vi "Set BBM Vacuum.vi"(6 "On/Off":bool, 8 "error in (no error)":errorcluster, 9 "Slot Number":u32, 10 "Chuck Number":u32, 11 "Gantry Class in":refnum<class "Gantry Class.lvclass">) -> (0 "error out":errorcluster, 3 "Gantry Class out":refnum<class "Gantry Class.lvclass">)   [LabVIEW 2011, in "Gantry Class.lvclass"]
uses:
  Gantry Class.lvclass
  WorkTable Class/WorkTable Class.lvclass
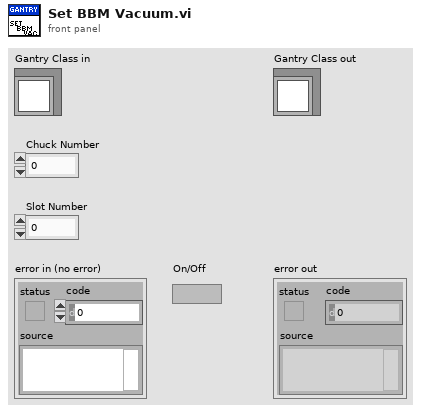
[diagram p1: front panel]
types:
  T1 = typedef "Worktable_BBM Slot.ctl" = cluster{"BBM Slot State":enum16{"Empty", "Unglued", "Stamped", "PartOnTop", "Weighted", "Unpotted", "Potted"}, "BBM Type":enum16{"BBM", "GlassSlide"}, "HDI Type":enum16{"HDI", "Polyimide"}, "Vacuum Channel":u8, "Location/Orientation BBM":T2, "Location/Orientation HDI":T2}
  T2 = typedef "Position_Orientation.ctl" = cluster{"Center":refnum<class "Vec3d Class.lvclass">, "Orientation":refnum<class "Orient3d Class.lvclass">}
  T3 = cluster{"BBM Chucks":cluster{"BBM Slots":T1[]}[]}
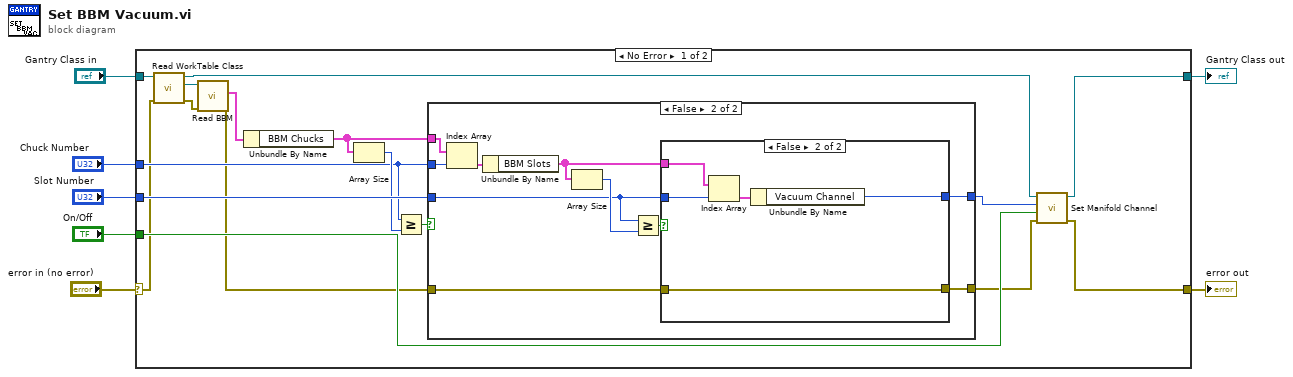
[diagram p0: block diagram]
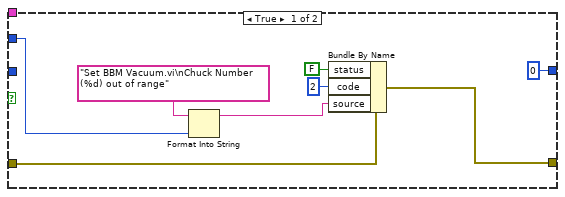
[diagram p2: hidden frame]
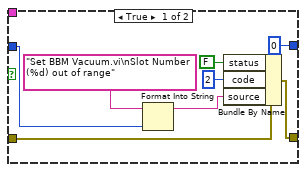
[diagram p3: hidden frame]
diagram:
  n1 = case shown="No Error" "error in (no error)" {
    selector: "error in (no error)" -> [w9 w57]
    tunnel: [w11 w57] -> w6
    tunnel: [w12 w56] -> w4
    tunnel: "Gantry Class in" -> [w24 w56]
    tunnel: "Chuck Number" -> [w18 _]
    tunnel: "Slot Number" -> [w21 _]
    tunnel: "On/Off" -> [w15 _]
    frame No Error {
      n2 = call-dynamic "Read WorkTable Class.vi"("error in"=w9, "Gantry Class in"=w24) -> ("error out"=w10:errorcluster, "WorkTable Class.lvclass"=w23:refnum<class "WorkTable Class.lvclass">, "Gantry Class out"=w13:refnum<class "Gantry Class.lvclass">)  [unwired: 7 in]
      n3 = call-dynamic "Read BBM.vi"("error in (no error)"=w10, "WorkTable Class in"=w23) -> ("error out"=w8:errorcluster, "BBM"=w22:T3)  [unwired: 7 in, 1 out]
      n4 = Unbundle By Name(w22) -> ("BBM Chucks"=w20:cluster{"BBM Slots":T1[]}[])
      n5 = Array Size(array=w20) -> (size(s)=w19:i32)
      n6 = Greater Or Equal?(x=w18, y=w19) -> (x >= y?=w17:bool)
      n7 = case shown="False" w17 {
        tunnel: w18 -> [w28 w42]
        tunnel: w21 -> [_ w36]
        tunnel: w20 -> [_ w40]
        tunnel: w8 -> [w25 w35]
        tunnel: [w27 w34] -> w14
        tunnel: [u8 0 ("Vacuum Channel") w33] -> w16
        frame True {
          n8 = Format Into String(format string="Set BBM Vacuum.vi\nChuck Number (%d) out of range" ("source"), w28) -> (resulting string=w29:string)  [unwired: 2 in, 1 out]
          n9 = Bundle By Name(cluster=w25, "status"=FALSE, "code"=2, "source"=w29) -> (w27:errorcluster)
        }
        frame False {
          n10 = Index Array(array=w40, index=w42) -> (element=w41:cluster{"BBM Slots":T1[]})
          n11 = Unbundle By Name(w41) -> ("BBM Slots"=w37:T1[])
          n12 = Array Size(array=w37) -> (size(s)=w39:i32)
          n13 = Greater Or Equal?(x=w36, y=w39) -> (x >= y?=w38:bool)
          n14 = case shown="False" w38 {
            tunnel: w37 -> [_ w55]
            tunnel: w36 -> [w46 w54]
            tunnel: w35 -> [w45 w51]
            tunnel: [w44 w51] -> w34
            tunnel: [u8 0 ("Vacuum Channel") w52] -> w33
            frame True {
              n15 = Format Into String(format string="Set BBM Vacuum.vi\nSlot Number (%d) out of range" ("source"), w46) -> (resulting string=w47:string)  [unwired: 2 in, 1 out]
              n16 = Bundle By Name(cluster=w45, "status"=FALSE, "code"=2, "source"=w47) -> (w44:errorcluster)
            }
            frame False {
              n17 = Index Array(array=w55, index=w54) -> (element=w53:T1)
              n18 = Unbundle By Name(w53) -> ("Vacuum Channel"=w52:u8)
            }
          }
        }
      }
      n19 = call-dynamic "Set Manifold Channel.vi"("error in (no error)"=w14, "On/Off"=w15, "Manifold Channel"=w16, "Gantry Class in"=w13) -> ("error out"=w11:errorcluster, "Gantry Class out"=w12:refnum<class "Gantry Class.lvclass">)  [unwired: 6 in]
    }
    frame Error {
    }
  }
  "error out" <- w6
  "Gantry Class out" <- w4
